vi "Reset VeriStand as Startup.vi"() -> ()   [LabVIEW 2014]
doc: "This VI is meant to be run from the VeriStand context. It queries the active system definition and ensures that VeriStand is set to be the startup executable on each of those targets."
uses:
  <vilib>/Utility/sysdir.llb/System Directory Type.ctl
  subVIs/Target Data Global.vi
  <vilib>/WebDAVClient/Advanced/Get File.vi
  <vilib>/WebDAVClient/Advanced/Put File.vi
  <vilib>/nisyscfg/Close (System).vi
  <vilib>/WebDAVClient/NI_WebDAV.lvlib
  <vilib>/nisyscfg/nisyscfg.lvlib
panel:
  out "Execution Log":string caption="Execution Log:"
  out "Waiting Lights":T1
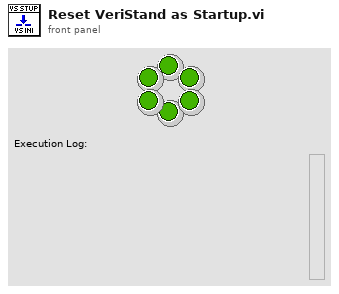
[diagram p1: front panel]
types:
  T1 = cluster{"wait 1":bool, "wait 2":bool, "wait 3":bool, "wait 4":bool, "wait 5":bool, "wait 6":bool}
  T2 = cluster{"OperatingSystem":string, "IPAddress":string}[]
  T3 = typedef "Target Specific Data.ctl" = cluster{"VS EXE Dir Uri":string, "ini or conf uri":string, "ini or conf name":string, "VS EXE Path":string}
  T4 = typedef "System Directory Type.ctl" = i32
  T5 = typedef "NI_WebDAV.lvlib/SessionHandle.ctl" = refnum<k1>
  T6 = cluster{"[0]":bool, "[1]":bool, "[2]":bool, "[3]":bool, "[4]":bool, "[5]":bool}
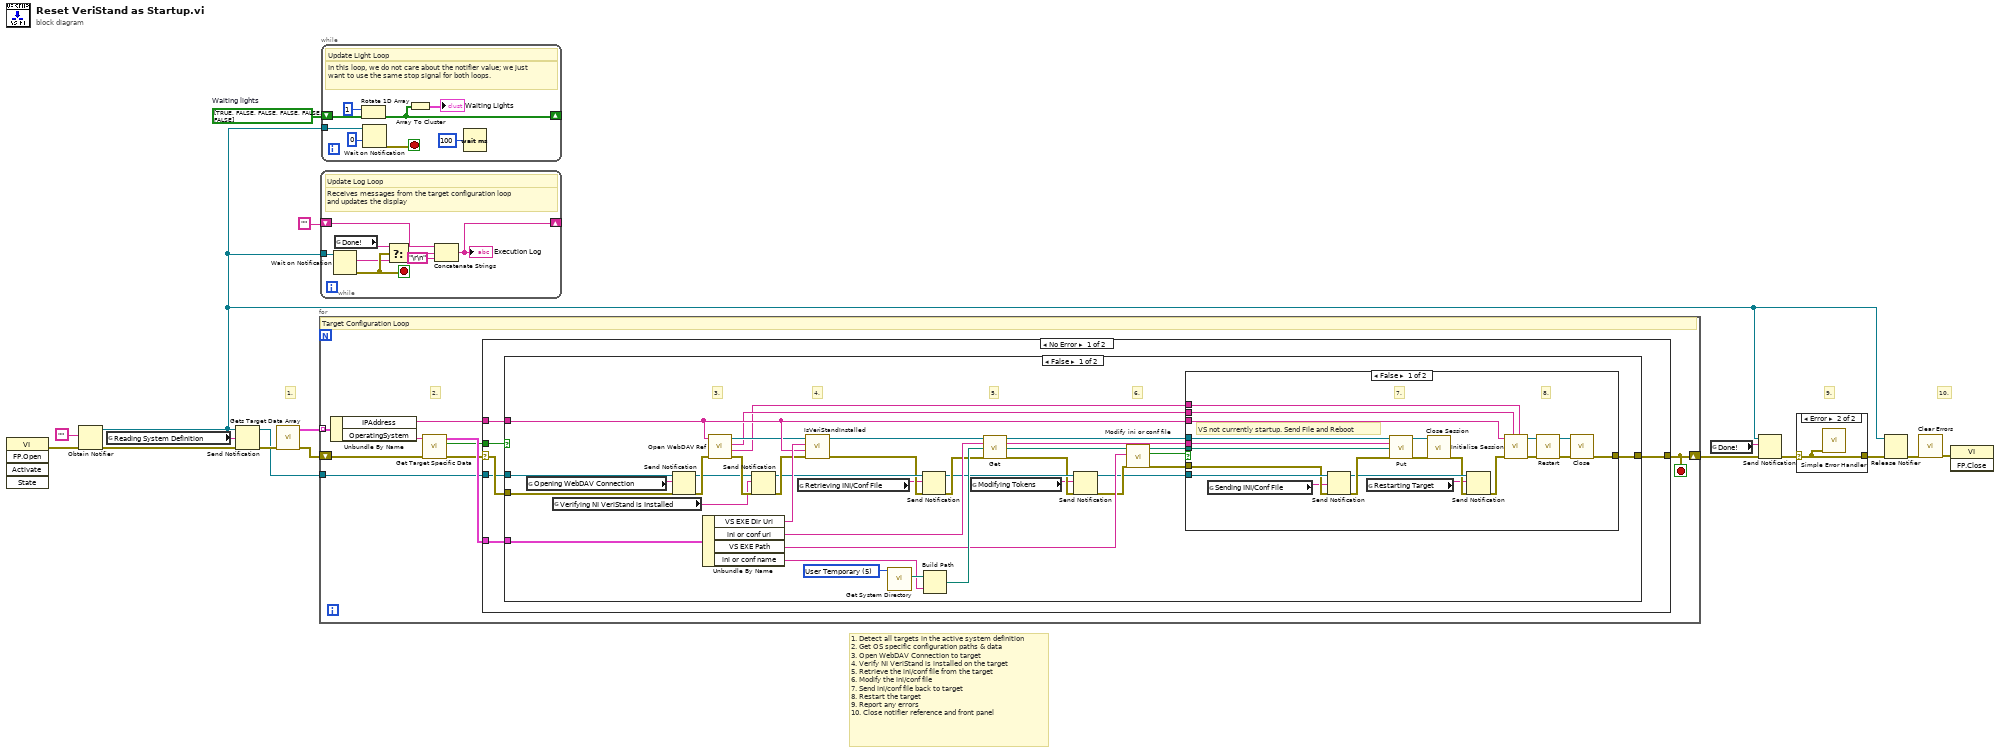
[diagram p0: block diagram]
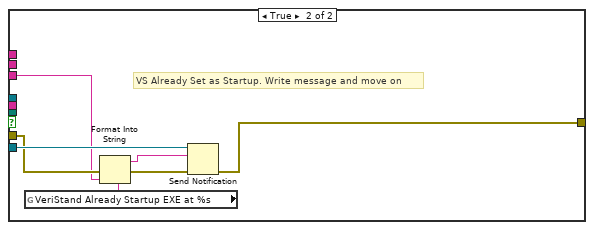
[diagram p2: hidden frame]
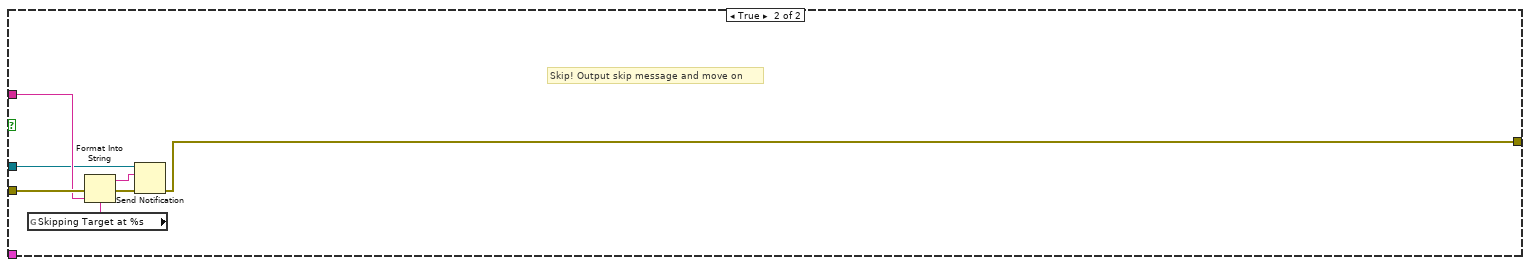
[diagram p3: hidden frame]
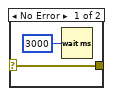
[diagram p5: hidden frame]
diagram:
  w15 = bool[] [TRUE, FALSE, FALSE, FALSE, FALSE, FALSE]  # Waiting lights
  # "10."
  # "9."
  # "1."
  # "1. Detect all targets in the active system definition\n2. Get OS specific configuration paths & data\n3. Open WebDAV Connection to target\n4. Verify NI VeriStand is installed on the target\n5. Retrieve the ini/conf file from the target\n6. Modify the ini/conf file\n7. Send ini/conf file back to target\n8. Restart the target\n9. Report any errors\n10. Close notifier reference and front panel"
  n1 = invoke class="VI" method="FP.Open"() -> (error out=w7:errorcluster)  [unwired: 5 in, 4 out]
  n2 = Obtain Notifier(notification data type="", error in (no error)=w7) -> (notifier out=w1:refnum<notifier>, error out=w13:errorcluster)  [unwired: 2 in, 1 out]
  n3 = global read "Target Data Global.vi" "Reading System Definition"() -> (w6:string)
  n4 = Send Notification(notification=w6, notifier=w1, error in (no error)=w13) -> (notifier out=w8:refnum<notifier>, error out=w11:errorcluster)
  n5 = call "Gets Target Data Array.vi"("error in (no error)"=w11) -> ("error out"=w9:errorcluster, "All Targets Data"=w10:T2)  [unwired: 9 in]
  n6 = for {
    tunnel: w10 -> [w26] mode=indexing
    shift-right: [w23] -> w3
    shift-left: w9 -> [w24]
    tunnel: w8 -> [w20]
    stop <- w23 stop-if-true
    # "2."
    # "Target Configuration Loop"
    n7 = Unbundle By Name(w26) -> ("IPAddress"=w22:string, "OperatingSystem"=w25:string)
    n8 = call "Get Target Specific Data.vi"("error in (no error)"=w24, "Operating System"=w25) -> ("error out"=w19:errorcluster, "Skip?"=w18:bool, "Target Specific Data"=w21:T3)  [unwired: 7 in]
    n9 = case shown="No Error" w19 {
      selector: w19 -> [w31 w104]
      tunnel: [w28 w104] -> w23
      tunnel: w22 -> [w30 _]
      tunnel: w21 -> [w32 _]
      tunnel: w20 -> [w29 _]
      tunnel: w18 -> [w27 _]
      frame No Error {
        n10 = case shown="False" w27 {
          tunnel: w32 -> [w68 _]
          tunnel: w31 -> [w56 w102]
          tunnel: w30 -> [w45 w101]
          tunnel: w29 -> [w40 w100]
          tunnel: [w34 w97] -> w28
          frame False {
            w65 = T4 5 items=["User Home"=0, "User Desktop"=1, "User Documents"=2, "User Application Data"=3, "User Preferences"=4, "User Temporary"=5, "Public Documents"=6, "Public Application Data"=7, "Public Preferences"=8, "Public Cache"=13, "System Core Libraries"=9, "System Installed Libraries"=10, "Application Files"=11, "Boot Volume Root"=12] ("system directory type")
            # "6."
            # "5."
            # "4."
            # "3."
            n11 = global read "Target Data Global.vi" "Opening WebDAV Connection"() -> (w38:string)
            n12 = global read "Target Data Global.vi" "Verifying NI VeriStand is Installed"() -> (w37:string)
            n13 = Send Notification(notification=w38, notifier=w40, error in (no error)=w56) -> (notifier out=w39:refnum<notifier>, error out=w55:errorcluster)
            n14 = Unbundle By Name(w68) -> ("VS EXE Dir Uri"=w67:string, "ini or conf uri"=w57:string, "VS EXE Path"=w59:string, "ini or conf name"=w63:string)
            n15 = call "Open WebDAV Ref.vi"("error in (no error)"=w55, "IPAddress"=w45) -> ("error out"=w43:errorcluster, "Password Output"=w41:string, "Username Output"=w42:string, "Refnum out"=w44:T5)  [unwired: 6 in]
            n16 = Send Notification(notification=w37, notifier=w39, error in (no error)=w43) -> (notifier out=w53:refnum<notifier>, error out=w54:errorcluster)
            n17 = global read "Target Data Global.vi" "Retrieving INI/Conf File"() -> (w36:string)
            n18 = call "IsVeriStandInstalled.vi"("error in (no error)"=w54, "Target IP Address"=w45, "VS EXE Install Dir Uri"=w67, "WebDav Ref In"=w44) -> ("error out"=w52:errorcluster, "WebDav Ref Out"=w64:T5)  [unwired: 6 in]
            n19 = call <vilib>:"Get System Directory.vi"("system directory type"=w65) -> ("system directory"=w66:path)  [unwired: 10 in]
            n20 = Send Notification(notification=w36, notifier=w53, error in (no error)=w52) -> (notifier out=w50:refnum<notifier>, error out=w51:errorcluster)
            n21 = Build Path(base path=w66, name or relative path=w63) -> (appended path=w62:path)
            n22 = global read "Target Data Global.vi" "Modifying Tokens"() -> (w35:string)
            n23 = call-poly <vilib>:"Get.vi"("session handle"=w64, "relative uri"=w57, "local file path"=w62, "error in (no error)"=w51) -> ("session handle out"=w61:T5, "local file path out"=w60:path, "error out"=w49:errorcluster)  [unwired: 9 in]
            n24 = Send Notification(notification=w35, notifier=w50, error in (no error)=w49) -> (notifier out=w47:refnum<notifier>, error out=w48:errorcluster)
            n25 = call "Modify ini or conf file.vi"("error in (no error)"=w48, "VS RT EXE Path"=w59, "Local Path to ini or conf file"=w60) -> ("error out"=w46:errorcluster, "VS Already Set as Startup?"=w33:bool, "Dup Path to ini or conf file"=w58:path)  [unwired: 6 in]
            n26 = case shown="False" w33 {
              tunnel: w61 -> [w83 _]
              tunnel: w58 -> [w82 _]
              tunnel: w57 -> [w81 _]
              tunnel: w47 -> [w80 w96]
              tunnel: w46 -> [w79 w94]
              tunnel: w45 -> [w74 w91]
              tunnel: w42 -> [w73 _]
              tunnel: w41 -> [w72 _]
              tunnel: [w69 w95] -> w34
              frame False {
                # "VS not currently startup. Send File and Reboot"
                # "8."
                # "7."
                n27 = global read "Target Data Global.vi" "Sending INI/Conf File"() -> (w71:string)
                n28 = Send Notification(notification=w71, notifier=w80, error in (no error)=w79) -> (notifier out=w77:refnum<notifier>, error out=w78:errorcluster)
                n29 = global read "Target Data Global.vi" "Restarting Target"() -> (w70:string)
                n30 = call-poly <vilib>:"Put.vi"("session handle"=w83, "relative uri"=w81, "local file path"=w82, "error in (no error)"=w78) -> ("session handle out"=w85:T5, "error out"=w84:errorcluster)  [unwired: 9 in, 1 out]
                n31 = call <vilib>:"Close Session.vi"("session handle"=w85, "error in (no error)"=w84) -> ("error out"=w76:errorcluster)  [unwired: 13 in]
                n32 = Send Notification(notification=w70, notifier=w77, error in (no error)=w76) -> (error out=w75:errorcluster)  [unwired: 1 out]
                n33 = call <vilib>:"Initialize Session.vi"("Password"=w72, "User Name"=w73, "error in (no error)"=w75, "Target (localhost)"=w74) -> ("error out"=w87:errorcluster, "Session out"=w86:refnum<k21>)  [unwired: 6 in]
                n34 = call <vilib>:"Restart.vi"("error in (no error)"=w87, "Session in"=w86) -> ("error out"=w88:errorcluster, "Session out"=w89:refnum<k21>)  [unwired: 7 in, 1 out]
                n35 = call-poly <vilib>:"Close.vi"("error in (no error)"=w88, "Session in"=w89) -> ("error out"=w69:errorcluster)  [unwired: 9 in]
              }
              frame True {
                # "VS Already Set as Startup. Write message and move on"
                n36 = global read "Target Data Global.vi" "VeriStand Already Startup EXE at %s"() -> (w92:string)
                n37 = Format Into String(format string=w92, error in=w94, w91) -> (resulting string=w90:string, error out=w93:errorcluster)  [unwired: 1 in]
                n38 = Send Notification(notification=w90, notifier=w96, error in (no error)=w93) -> (error out=w95:errorcluster)  [unwired: 1 out]
              }
            }
          }
          frame True {
            # "Skip! Output skip message and move on"
            n39 = global read "Target Data Global.vi" "Skipping Target at %s"() -> (w103:string)
            n40 = Format Into String(format string=w103, error in=w102, w101) -> (resulting string=w98:string, error out=w99:errorcluster)  [unwired: 1 in]
            n41 = Send Notification(notification=w98, notifier=w100, error in (no error)=w99) -> (error out=w97:errorcluster)  [unwired: 1 out]
          }
        }
      }
      frame Error {
        # "Error or Skipping"
      }
    }
  }
  n42 = while {
    tunnel: w1 -> [w112]
    shift-right: [w105] -> _
    shift-left: "" -> [w108]
    stop <- w111 stop-if-true
    # "Receives messages from the target configuration loop       \nand updates the display"
    # "Update Log Loop"
    n43 = Wait on Notification(notifier=w112) -> (notification=w110:string, error out=w111:errorcluster)  [unwired: 3 in, 2 out]
    n44 = global read "Target Data Global.vi" "Done!"() -> (w109:string)
    n45 = Select(t=w109, s=w111, f=w110) -> (s? t:f=w107:string)
    n46 = Concatenate Strings(w108, w107, "\r\n") -> (w105:string)
    "Execution Log" <- w105
  }
  n47 = while {
    shift-right: [w114] -> _
    shift-left: w15 -> [w116]
    tunnel: w1 -> [w118]
    stop <- w120 stop-if-true
    # "In this loop, we do not care about the notifier value; we just want to use the same stop signal for both loops."
    # "Update Light Loop"
    n48 = Rotate 1D Array(1:w116, 2:1 ("n")) -> (0:w114:bool[])
    n49 = Wait on Notification(notifier=w118, timeout in ms (-1)=0) -> (error out=w120:errorcluster)  [unwired: 2 in, 3 out]
    n50 = Array To Cluster(array=w114) -> (cluster=→"Waiting Lights":T6)
    n51 = Wait (ms)(milliseconds to wait=u32 100) -> ()  [unwired: 1 out]
  }
  n52 = global read "Target Data Global.vi" "Done!"() -> (w4:string)
  n53 = Send Notification(notification=w4, notifier=w1, error in (no error)=w3) -> (error out=w2:errorcluster)  [unwired: 1 out]
  n54 = case shown="Error" w2 {
    tunnel: [w122 w123] -> w12
    selector: w2 -> [w122 w123]
    frame No Error {
      n55 = Wait (ms)(milliseconds to wait=u32 3000) -> ()  [unwired: 1 out]
    }
    frame Error {
      n56 = call <vilib>:"Simple Error Handler.vi"("error in (no error)"=w123) -> ()  [unwired: 4 in, 5 out]
    }
  }
  n57 = Release Notifier(notifier=w1, error in (no error)=w12) -> (error out=w17:errorcluster)  [unwired: 1 in, 2 out]
  n58 = call <vilib>:"Clear Errors.vi"("error in (no error)"=w17) -> ("error out"=w14:errorcluster)  [unwired: 5 in, 1 out]
  n59 = invoke class="VI" method="FP.Close"(error in=w14) -> ()  [unwired: 2 in, 3 out]
